vi "Problema3_3.vi"() -> ()   [LabVIEW 2020]
panel:
  in  "Y":dbl
  in  "X":dbl
  out "XY Graph":cluster{"Y":dbl[], "Y":dbl[]}[](graph)
  # "Radio en X"
  # "Ya que la ecala se modifica y no es cuadrada, por lo mismo la elipce se ve mas circular de lo que es"
  # "Radio en Y"
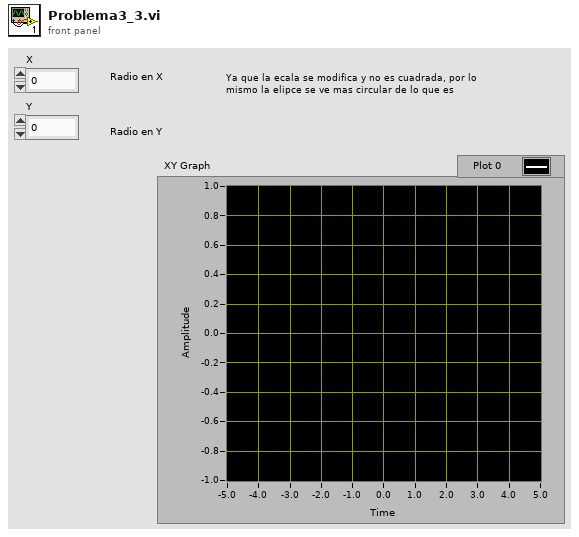
[diagram p1: front panel]
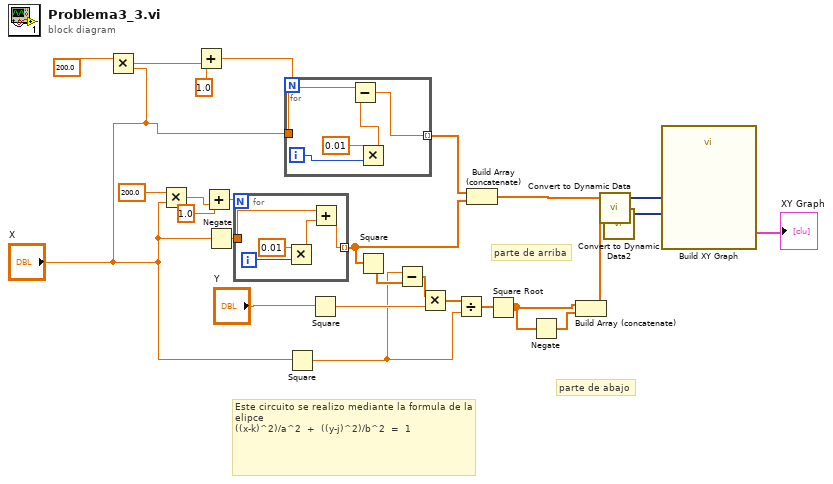
[diagram p0: block diagram]
diagram:
  # "Este circuito se realizo mediante la formula de la elipce \n((x-k)^2)/a^2  +  ((y-j)^2)/b^2  =  1"
  # "parte de abajo"
  # "parte de arriba"
  n1 = Multiply(x=200.0, y="X") -> (x*y=w6:dbl)
  n2 = Multiply(x=200.0, y="X") -> (x*y=w13:dbl)
  n3 = Add(x=1.0, y=w6) -> (x+y=w7:dbl)
  n4 = Add(x=1.0, y=w13) -> (x+y=w14:dbl)
  n5 = Negate(x="X") -> (-x=w24:dbl)
  n6 = for {
    N: w14 -> [_]
    tunnel: w24 -> [w31]
    tunnel: [w30] -> w8 mode=indexing
    i -> [w28]
    n7 = Multiply(x=0.01, y=w28) -> (x*y=w27:dbl)
    n8 = Add(x=w31, y=w27) -> (x+y=w30:dbl)
  }
  n9 = for {
    N: w7 -> [_]
    tunnel: "X" -> [w36]
    tunnel: [w35] -> w2 mode=indexing
    i -> [w32]
    n10 = Multiply(x=0.01, y=w32) -> (x*y=w34:dbl)
    n11 = Subtract(x=w36, y=w34) -> (x-y=w35:dbl)
  }
  n12 = Square(x="X") -> (x^2=w15:dbl)
  n13 = Square(x="Y") -> (x^2=w20:dbl)
  n14 = Square(x=w8) -> (x^2=w17:dbl[])
  n15 = Subtract(x=w15, y=w17) -> (x-y=w18:dbl[])
  n16 = Multiply(x=w18, y=w20) -> (x*y=w19:dbl[])
  n17 = Divide(x=w19, y=w15) -> (x/y=w22:dbl[])
  n18 = Build Array (concatenate)(w2, w8) -> (w1:dbl[])
  n19 = Square Root(x=w22) -> (sqrt(x)=w10:dbl[])
  n20 = Negate(x=w10) -> (-x=w11:dbl[])
  n21 = Build Array (concatenate)(w10, w11) -> (w9:dbl[])
  n22 = call "Convert to Dynamic Data"("Array"=w1) -> ("Dynamic Data Type"=w23:dynamicdata)  [unwired: 3 in]
  n23 = call "Convert to Dynamic Data2"("Array"=w9) -> ("Dynamic Data Type"=w16:dynamicdata)  [unwired: 3 in]
  n24 = call "Build XY Graph"("Y Input"=w16, "X Input"=w23) -> ("XY Graph"=→"XY Graph":cluster{"X":dbl[], "Y":dbl[]}[])  [unwired: 8 in, 1 out]
